vi "proba_ui_kor_draw.vi"() -> ()   [LabVIEW 2012]
panel:
  out "Joy":picture
types:
  T1 = cluster{"Width":u16, "Style":enum32{"Solid", "Dash", "Dot", "DashDot", "DashDotDot"}}
  T2 = cluster{"left":i16, "top":i16, "right":i16, "bottom":i16}
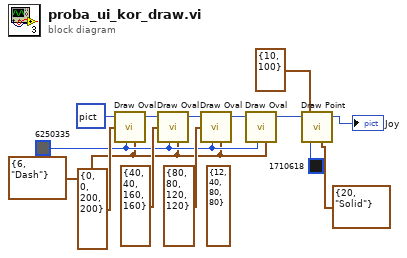
[diagram p0: block diagram]
diagram:
  w8 = u32 6250335
  (unwired) T2 {"left"=12, "top"=40, "right"=80, "bottom"=80} ("rect")
  w6 = T1 {"Width"=6, "Style"=enum."Dash"} ("pen")
  n1 = call <vilib>:"Draw Oval.vi"("picture"=picture data[5B], "rect"=T2 {"left"=0, "top"=0, "right"=200, "bottom"=200}, "color(black)"=w8, "pen"=w6) -> ("new picture"=w14:picture)  [unwired: 5 in]
  n2 = call <vilib>:"Draw Oval.vi"("picture"=w14, "rect"=T2 {"left"=40, "top"=40, "right"=160, "bottom"=160}, "color(black)"=w8, "pen"=w6) -> ("new picture"=w11:picture)  [unwired: 5 in]
  n3 = call <vilib>:"Draw Oval.vi"("picture"=w11, "rect"=T2 {"left"=80, "top"=80, "right"=120, "bottom"=120}, "color(black)"=w8, "pen"=w6) -> ("new picture"=w9:picture)  [unwired: 5 in]
  n4 = call <vilib>:"Draw Oval.vi"("picture"=w9, "color(black)"=w8, "pen"=w6) -> ("new picture"=w4:picture)  [unwired: 6 in]
  n5 = call <vilib>:"Draw Point.vi"("picture"=w4, "point(x,y)"=cluster{"x":i16, "y":i16} {"x"=10, "y"=100}, "color(black)"=u32 1710618, "pen"=T1 {"Width"=20, "Style"=enum."Solid"}) -> ("new picture"=→"Joy":picture)  [unwired: 5 in]
